vi "Count Devices.vi"(8 "error in (no error)":errorcluster) -> (0 "error out":errorcluster, 2 "Number of Devices":i32)   [LabVIEW 2019, in "D2XX-lv.lvlib"]
doc: "Returns the <b>Number of Devices</b> connected."
uses:
  D2XX-lv.lvlib
  <instrlib>/_D2XX/D2XX/D2XX.lvlib
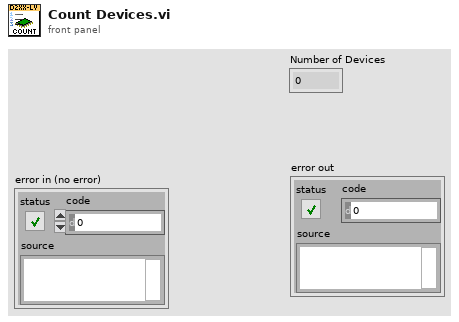
[diagram p1: front panel]
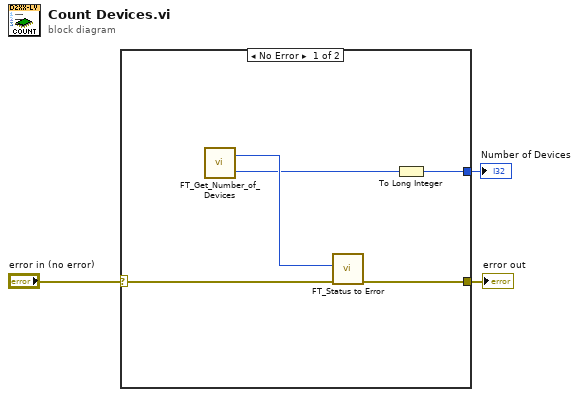
[diagram p0: block diagram]
diagram:
  n1 = case shown="No Error" "error in (no error)" {
    selector: "error in (no error)" -> [w8 w9]
    tunnel: [w7 w9] -> w2
    tunnel: [w4 _] -> w1
    frame No Error {
      n2 = call <instrlib>:"FT_Get_Number_of_Devices.vi"() -> ("Number of Devices"=w5:u16, "FT_Status"=w6:u32)
      n3 = call "FT_Status to Error.vi"("error in (no error)"=w8, "FT_Status"=w6) -> ("error out"=w7:errorcluster)  [unwired: 9 in]
      n4 = To Long Integer(number=w5) -> (32bit integer=w4:i32)
    }
    frame Error {
    }
  }
  "error out" <- w2
  "Number of Devices" <- w1
